vi "I2C_ID_SetMotor.vi"() -> ()   [LabVIEW 2017]
uses:
  <vilib>/myRIO/Common/Instrument Driver Framework/myRIO v1.0/UART/vis/myRIO v1.0 Close UART.vi
  <vilib>/myRIO/Common/Instrument Driver Framework/Utilities/vis/FPGA Ref Manager.vi
  <vilib>/myRIO/Common/Instrument Driver Framework/myRIO v1.0/myRIO v1.0 Reset FPGA.vi
  <vilib>/myRIO/Common/Instrument Driver Framework/myRIO v1.0/IRQ/vis/myRIO v1.0 IRQ Info FGV.vi
  <vilib>/myRIO/Common/Instrument Driver Framework/myRIO v1.0/IRQ/vis/myRIO v1.0 Timer IRQ Info FGV.vi
  <vilib>/myRIO/Common/Instrument Driver Framework/myRIO v1.0/IRQ/vis/myRIO v1.0 ISR Agent.vi
  <vilib>/myRIO/Instrument Drivers/Utilities/Utilities.lvlib
panel:
  out "error out":errorcluster
  in  "New ID# / I2C Address":u8=1
  in  "Current ID#  / I2C Address":u8=1 min=1 max=4
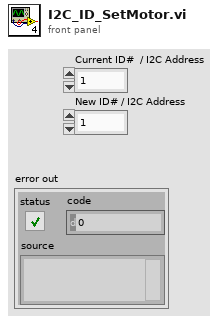
[diagram p1: front panel]
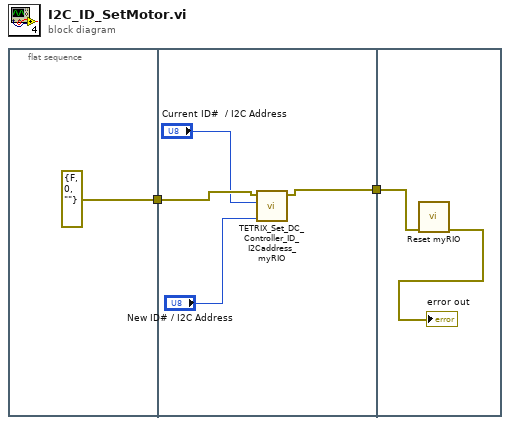
[diagram p0: block diagram]
diagram:
  n1 = flat-sequence {
    tunnel: [errorcluster {"status"=FALSE, "code"=0, "source"=""} ("error constant")] -> w2
    tunnel: w2 -> [w7]
    tunnel: [w4] -> w1
    tunnel: w1 -> [w9]
    frame #0 {
    }
    frame #1 {
      n2 = call <vilib>:"TETRIX_Set_DC_Controller_ID_I2Caddress_myRIO.vi"("New ID# / I2C Address"="New ID# / I2C Address", "Current ID#  / I2C Address"="Current ID#  / I2C Address", "Error/Flow In"=w7) -> ("Error/Flow Out"=w4:errorcluster)  [unwired: 4 in]
    }
    frame #2 {
      n3 = call <vilib>:"Reset myRIO.vi"("error in (no error)"=w9) -> ("error out"=→"error out":errorcluster)  [unwired: 10 in]
    }
  }
